vi "Core Action.vi"(8 "error in (no error)":errorcluster, 10 "SECS-II Class":refnum<class "SECS-II Class.lvclass">, 11 "15-Process Program Request in":refnum<class "15-Process Program Request.lvclass">) -> (0 "error out":errorcluster, 2 "SECS-II Class Out":refnum<class "SECS-II Class.lvclass">, 3 "15-Process Program Request out":refnum<class "15-Process Program Request.lvclass">)   [LabVIEW 2020, in "SECS Scenarios.lvlib" / "15-Process Program Request.lvclass"]
uses:
  15-Process Program Request.lvclass
  D:/Dropbox/SECS/SECS_GEM v1.1.0/Com/SECS Scenarios/Scenarios Class/Scenarios Class.lvclass
  SECS Communication/SECS-II Class/SECS-II Class.lvclass
  SECS Communication/S7 Message Class/S7 Message Class.lvclass
  D:/Dropbox/SECS/SECS_GEM v1.1.0/Com/SECS Communication/SECS-II Class/SECS-II Class.lvclass
  Scenarios Class/Reply State.ctl
  Scenarios Class/Scenarios Class.lvclass/Scenarios Class.ctl
  SECS Communication/S7 Message Class/S7F6.ctl
  Scenarios Class/Write Reply State.vi
  Scenarios Class/Read HSMS Class.vi
  SECS Communication/HSMS Class/HSMS Class.lvclass
  Scenarios Class/Scenarios Class.lvclass
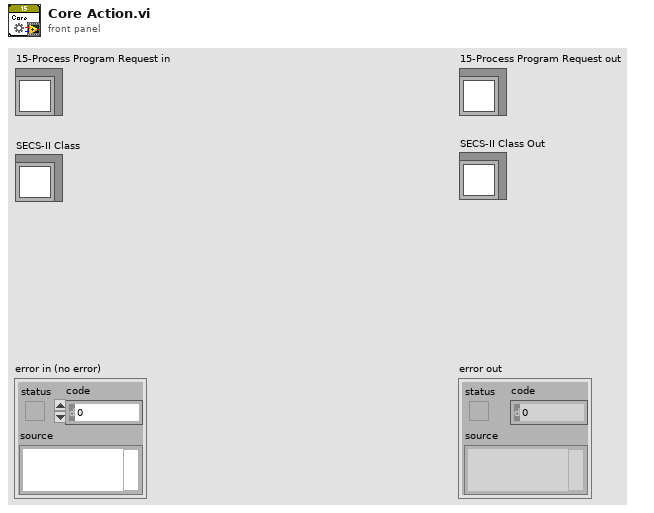
[diagram p1: front panel]
types:
  T1 = typedef "SECS Scenarios.lvlib/Scenarios Class.lvclass/Reply State.ctl" = enum16{"OK", "Illegal Data", "Unknown Stream", "Unknown Function", "Off-Line", "T3 Timeout", "Inner-Timeout"}
  T2 = typedef "SECS Communication.lvlib/S7 Message Class.lvclass/S7F6.ctl" = cluster{"PPID":string, "PPBODY":u8[]}
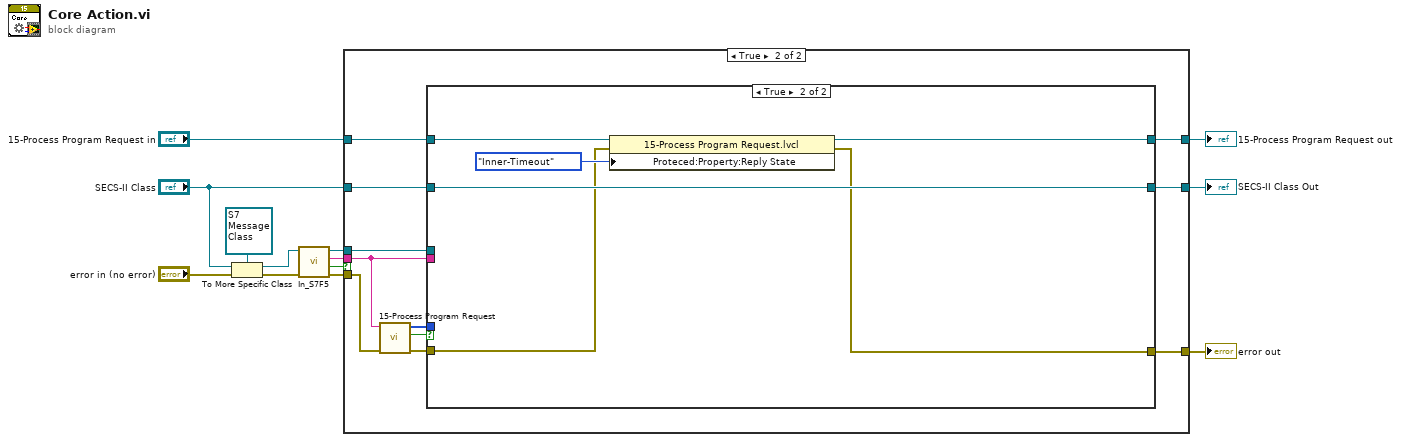
[diagram p0: block diagram]
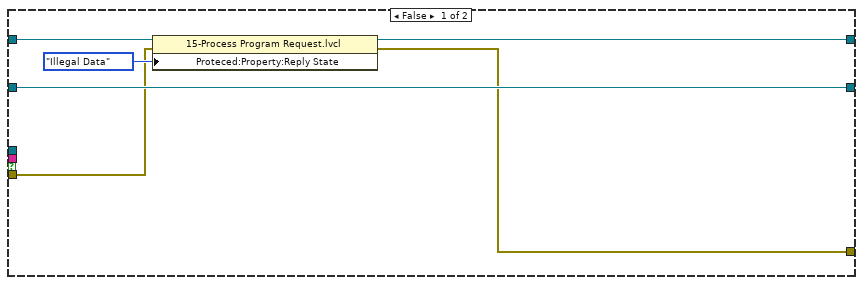
[diagram p2: hidden frame]
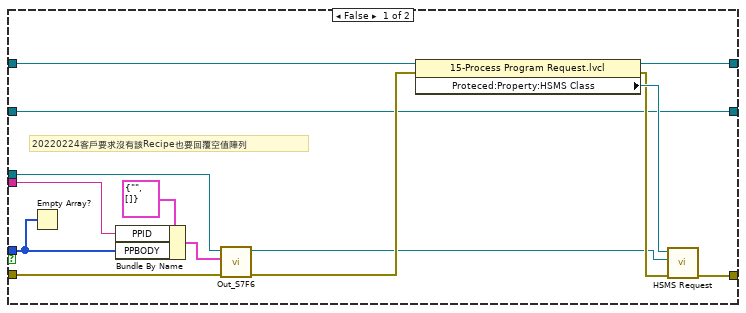
[diagram p3: hidden frame]
diagram:
  n1 = To More Specific Class(target class=refnum<class "S7 Message Class.lvclass"> refnum ("S7 Message Class in"), reference="SECS-II Class", error in="error in (no error)") -> (specific class reference=w10:refnum<class "S7 Message Class.lvclass">, error out=w11:errorcluster)
  n2 = call "In_S7F5.vi"("error in (no error)"=w11, "S7 Message Class in"=w10) -> ("error out"=w9:errorcluster, "OK?"=w1:bool, "PPID"=w6:string, "S7 Message Class out"=w8:refnum<class "S7 Message Class.lvclass">)  [unwired: 6 in]
  n3 = case shown="True" w1 {
    tunnel: w9 -> [w15 w30]
    tunnel: w8 -> [_ w26]
    tunnel: "15-Process Program Request in" -> [w19 w25]
    tunnel: w6 -> [_ w24]
    tunnel: [w14 w23] -> w5
    tunnel: [w18 w22] -> w4
    tunnel: "SECS-II Class" -> [w17 w21]
    tunnel: [w17 w20] -> w2
    frame False {
      n4 = property class="15-Process Program Request.lvcl"(reference=w19, error in=w15, "Proteced:Property:Reply State"=Reply_State."Illegal Data" ("Reply State")) -> (reference out=w18:refnum<class "15-Process Program Request.lvclass">, error out=w14:errorcluster)
    }
    frame True {
      n5 = call "15-Process Program Request.vi"("error in (no error)"=w30, "PPID"=w24) -> ("error out"=w29:errorcluster, "Timeout?"=w28:bool, "PPBODY"=w27:u8[])  [unwired: 7 in]
      n6 = case shown="True" w28 {
        tunnel: w25 -> [w44 w48]
        tunnel: w26 -> [w38 _]
        tunnel: [w41 w45] -> w23
        tunnel: [w40 w46] -> w22
        tunnel: w29 -> [w39 w47]
        tunnel: w27 -> [w33 _]
        tunnel: w24 -> [w37 _]
        tunnel: w21 -> [w34 w50]
        tunnel: [w34 w50] -> w20
        frame False {
          # "20220224客戶要求沒有該Recipe也要回覆空值陣列"
          n7 = Empty Array?(array=w33) -> ()  [unwired: 1 out]
          n8 = Bundle By Name(cluster=T2 {"PPID"="", "PPBODY"=[]} ("S7F6"), "PPID"=w37, "PPBODY"=w33) -> (w32:T2)
          n9 = call "Out_S7F6.vi"("error in (no error)"=w39, "S7F6"=w32, "S7 Message Class in"=w38) -> ("error out"=w36:errorcluster, "S7 Message Class out"=w35:refnum<class "S7 Message Class.lvclass">)  [unwired: 7 in]
          n10 = property class="15-Process Program Request.lvcl"(reference=w44, error in=w36) -> (reference out=w40:refnum<class "15-Process Program Request.lvclass">, error out=w42:errorcluster, "Proteced:Property:HSMS Class"=w43:refnum<class "HSMS Class.lvclass">)
          n11 = call "HSMS Request.vi"("error in (no error)"=w42, "SECS-II Class In"=w35, "HSMS Class in"=w43) -> ("error out"=w41:errorcluster)  [unwired: 7 in, 1 out]
        }
        frame True {
          n12 = property class="15-Process Program Request.lvcl"(reference=w48, error in=w47, "Proteced:Property:Reply State"=Reply_State."Inner-Timeout" ("Reply State")) -> (reference out=w46:refnum<class "15-Process Program Request.lvclass">, error out=w45:errorcluster)
        }
      }
    }
  }
  "error out" <- w5
  "15-Process Program Request out" <- w4
  "SECS-II Class Out" <- w2
